vi "OE1022D_Configure Harmonic.vi"(7 "OE1022D_Configure Harmonic":T1={"Harmonic 1"=1, "Harmonic 2"=1, "Channel"=1} {"Channel" items=["A"=1, "B"=2]; "Harmonic 2" min=1 max=32767; "Harmonic 1" min=1 max=32767}, 8 "Error in (no error)":errorcluster caption="error out（no error）", 9 "Remote Mode":u16(ring) items=["USB", "RS232", "GPIB"], 11 "VISA resource name":refnum<visa-resource-name>) -> (0 "Error out":errorcluster caption="error out", 1 "Output String":string, 3 "VISA resource  out":refnum<visa-resource-name>)   [LabVIEW 2011]
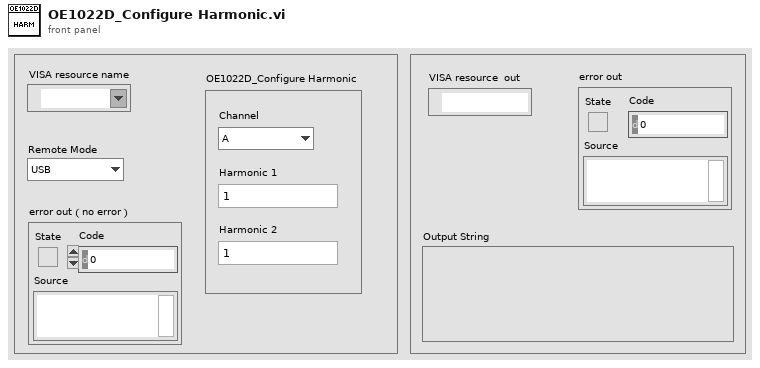
[diagram p1: front panel]
types:
  T1 = cluster{"Harmonic 1":u16, "Harmonic 2":u16, "Channel":u16}
  T2 = enum16{"ISRC", "IGND", "ICPL", "ILIN", "PHAS", "FMOD", "RSLP", "FREQ", "SWPT", "SLLM", "SULM", "SSLL", "SSLG", "STLM", "SWRM", "IRNG", "SENS", "RMOD", "OFLT", "OFSL", "SYNC", "DMOD", "HARM", "DARB", "SWVT", "SLVL", "SVLL", "SVUL", "SVSL", "SVSG", "SVTM", "SVRM", "RALL", "SNAP", "OUTP", "OAUX", "COUT", "CAUX", "COFP", "CEXP", "FPOP", "OEXP", "*IDN", "*RST", "OVLD", "INOV", "GNOV", "*PLL", "SSET", "RSET", "AGAN", "APHS", "ARSV", "ASCL", "EQCD", "EQCS", "SPED", "SRAT", "SLEN", "SSLE", "STRG", "SPRM", "STRD", "PAUS", "REST", "SPTS", "TRCA", "TEMP", "RSTU", "IHNZ", "DEQU", "SADD", "ARNG", "CSPE", "ISRCD", "IGNDD", "ICPLD", "ILIND", "PHASD", "FMODD", "RSLPD", "FREQD", "SWPTD", "SLLMD", "SULMD", "SSLLD", "SSLGD", "STLMD", "SWRMD", "SENSD", "RMODD", "OFLTD", "OFSLD", "SYNCD", "HARMD", "EQCDD", "EQCSD", "SNAPD", "OUTPD", "SWVTD", "SLVLD", "SVLLD", "SVULD", "SVSLD", "SVSGD", "SVTMD", "SVRMD", "SVDCD", "ARSVD", "AGAND", "APHSD", "ASCLD", "FPOPD", "CAUXD", "OEXPD", "SPEDD", "SRATD", "SLEND", "SSLED", "STRGD", "SPRMD", "STRDD", "PAUSD", "RESTD", "SPTSD", "TRCAD", "*IDND", "*RSTD", "INOVD", "GNOVD", "*PLLD", "SSETD", "RSETD"}
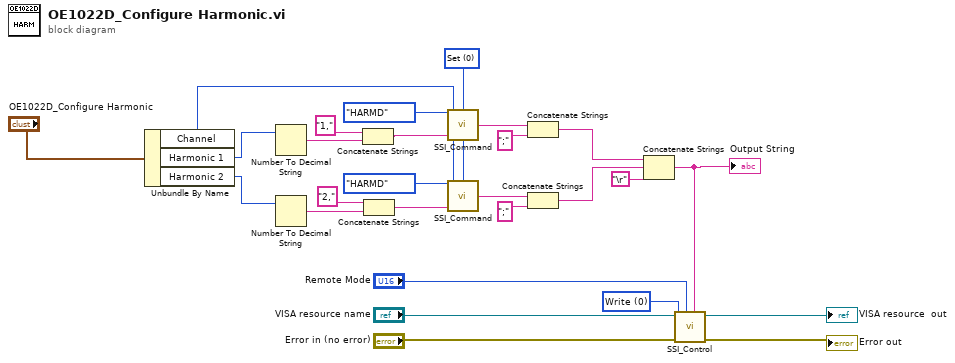
[diagram p0: block diagram]
diagram:
  w13 = u16 0 items=["Set", "Query"] ("Opera")
  w26 = u16 0 items=["Write", "Read"] ("Control")
  n1 = Unbundle By Name("OE1022D_Configure Harmonic") -> ("Channel"=w9:u16, "Harmonic 1"=w19:u16, "Harmonic 2"=w16:u16)
  n2 = Number To Decimal String(number=w19) -> (decimal integer string=w4:string)  [unwired: 1 in]
  n3 = Number To Decimal String(number=w16) -> (decimal integer string=w2:string)  [unwired: 1 in]
  n4 = Concatenate Strings("1," ("字符串"), w4) -> (w5:string)
  n5 = Concatenate Strings("2," ("字符串"), w2) -> (w3:string)
  n6 = call "SSI_Command.vi"("Opera"=w13, "Paramter"=w5, "channel"=w9, "Command Type"=T2."HARMD") -> ("Output string"=w7:string)
  n7 = call "SSI_Command.vi"("Opera"=w13, "Paramter"=w3, "channel"=w9, "Command Type"=T2."HARMD") -> ("Output string"=w8:string)
  n8 = Concatenate Strings(w7, ";") -> (w12:string)
  n9 = Concatenate Strings(w8, ";") -> (w11:string)
  n10 = Concatenate Strings(w12, w11, "\r") -> (w21:string)
  "Output String" <- w21
  n11 = call "SSI_Control.vi"("Write Buffer"=w21, "Remote Mode"="Remote Mode", "Error in (no error)"="Error in (no error)", "Control"=w26, "VISA resource name"="VISA resource name") -> ("Error out"=→"Error out":errorcluster, "VISA resource  out"=→"VISA resource  out":refnum<visa-resource-name>)  [unwired: 3 in, 2 out]
